vi "Read Measurements.vi"(8 "error in (no error)":errorcluster, 11 "PacificPowerSource in":refnum<class "PacificPowerSource.lvclass">) -> (0 "error out":errorcluster, 2 "BaseMeasurements":T1, 3 "PacificPowerSource out":refnum<class "PacificPowerSource.lvclass">)   [LabVIEW 2018, in "AcPwrPlugins.lvlib" / "PacificPowerSource.lvclass"]
uses:
  PacificPowerSource.lvclass
  TypeDefs/Measurements.ctl
  PacificPowerSource.lvclass/PacificPowerSource.ctl
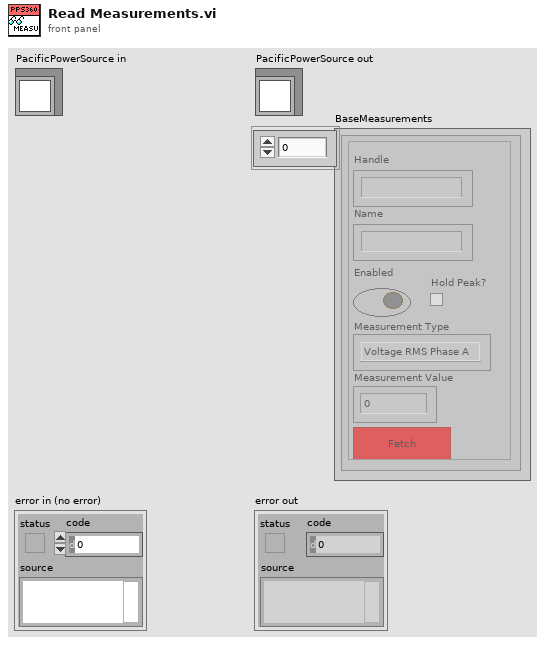
[diagram p1: front panel]
types:
  T1 = typedef "AcPwrPlugins.lvlib/PacificPowerSource.lvclass/Measurements.ctl" = cluster{"Handle":string, "Name":string, "Enabled":bool, "Measurement Value":dbl, "Measurement Type":enum16{"Voltage RMS Phase A", "Voltage RMS Phase B", "Voltage RMS Phase C", "Voltage RMS Phase A-B", "Voltage RMS Phase B-C", "Voltage RMS Phase C-A", "Current RMS Phase A", "Current RMS Phase B", "Current RMS Phase C", "Current Peak Phase A", "Current Peak Phase B", "Current Peak Phase C", "Current Crest Phase A", "Current Crest Phase B", "Current Crest Phase C", "KiloWatt Phase A", "KiloWatt Phase B", "KiloWatt Phase C", "KVA Phase A", "KVA Phase B", "KVA Phase C", "Power Factor A", "Power Factor B", "Power Factor C"}, "btnMeasFetch":bool, "Hold Peak?":bool}[]
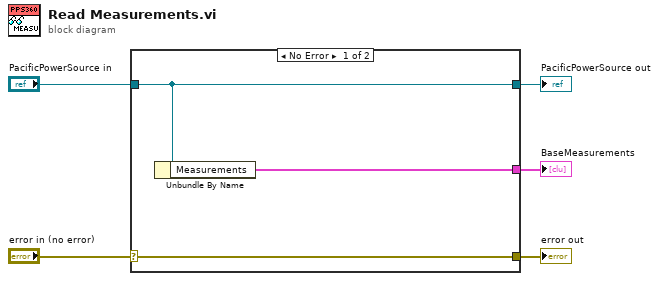
[diagram p0: block diagram]
diagram:
  n1 = case shown="No Error" "error in (no error)" {
    selector: "error in (no error)" -> [w8 w9]
    tunnel: [w8 w9] -> w4
    tunnel: [w7 w10] -> w2
    tunnel: "PacificPowerSource in" -> [w7 w10]
    tunnel: [w6 _] -> w1
    frame No Error {
      n2 = Unbundle By Name(w7) -> ("Measurements"=w6:T1)
    }
    frame Error {
    }
  }
  "error out" <- w4
  "PacificPowerSource out" <- w2
  "BaseMeasurements" <- w1
